vi "deadzone.vi"(2 "DeadZone":dbl, 3 "Input":dbl) -> (0 "Output":dbl)   [LabVIEW 2023]
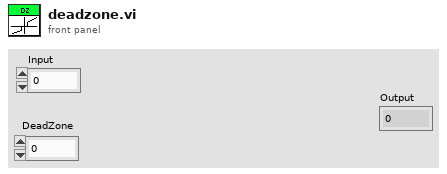
[diagram p1: front panel]
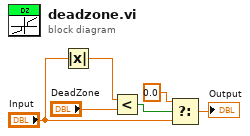
[diagram p0: block diagram]
diagram:
  n1 = Absolute Value(x="Input") -> (abs(x)=w4:dbl)
  n2 = Less?(x=w4, y="DeadZone") -> (x < y?=w5:bool)
  n3 = Select(t=0.0, s=w5, f="Input") -> (s? t:f=→"Output":dbl)
